vi "Live_Camram_Example_IMAQ.vi"() -> ()   [LabVIEW 2019]
doc: "A short program to demonstrate the fundamentals of control and image acquision with the pco.camera series. The program records a sequence of images, with \"live\" updating, until the \"StopRecording\" button is pressed. Use ctrl-H for more help on the individual controls and indicators.\n\nCopyright 2004, 2010 The Cooke Corporation."
uses:
  camera/Camera.lvclass
  pco.sdk/TimingControl/TimingControl.lvlib
panel:
  in  "Trigger":bool
  in  "data_format":T1(ring)=enum."Mono16"
  out "Image":T2(plugin-control)
  out "rawImage":u16[][](array[numeric])
  in  "Image Index":u32 max=9
  out "Recorded Images":u32
  in  "TriggerMode":T3(ring)
  in  "Quit":bool
  out "Error":errorcluster {"code" format="%x"}
  in  "Stop Record":bool
  out "Recording On":bool
  in  "roiY1":u64=2 min=1 max=1040 step=1
  in  "roiX1":u64=2 min=1 max=1392 step=1
  in  "roiY0":u64=1 min=1 max=1039 step=1
  in  "roiX0":u64=1 min=1 max=1391 step=1
  out "Image Height":u64
  out "Image Width":u64
  in  "segment":u16=1 caption="Segment" min=1 max=4
  in  "Exposure Time [s]":dbl=0.010000000000000002 min=1e-06 max=60.0 step=0.001
  # "This example demonstrates recording with live view for cameras with internal memory. \nDuring record, the latest transfered image is shown, after record is stopped, the images insisde the camera's ram can be addressed by index.\nNote that this example will not be fail save, i.e. doesnt react on errors, just handles them forward to the end\n\nUsage:\nSelect your required segment you want to record to, data format and the camera setup before you start the program.\nOnce started, the camera class will be initialized and images will be recorded and displayed automatically\nYou can stop the images by pressing stop record.\nAfter stopped, the image at the selected index will be read from the camera's RAM\nTo finish the program click on quit application, this will force an exit of the camera class\nYou can change your required ROI after and also during the record."
  # "pco.labview"
  # "Camera Setup"
  # "Recording Control"
  # "Parameters for image readout"
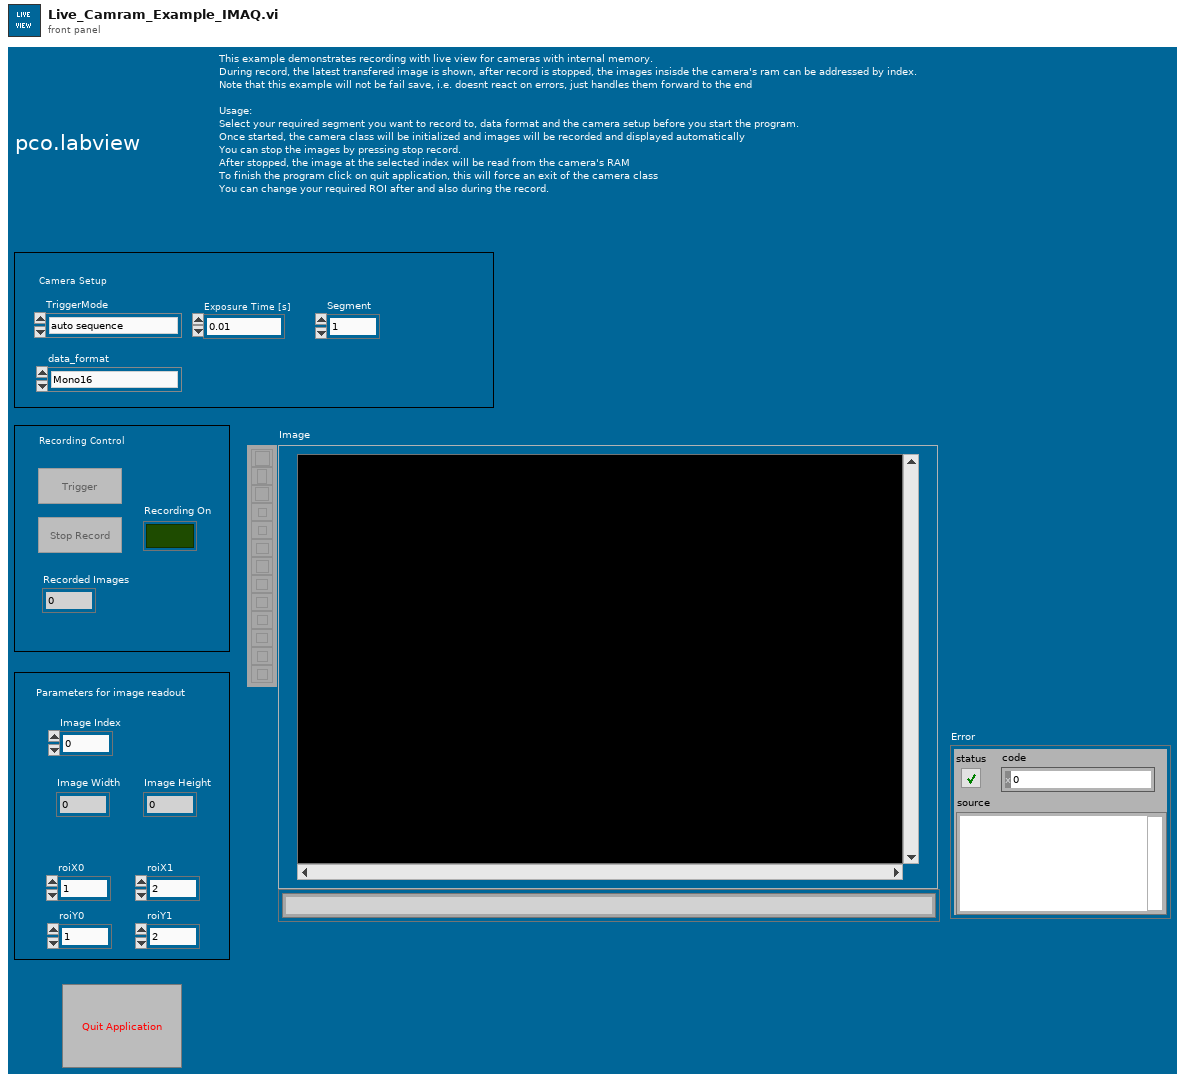
[diagram p1: front panel]
types:
  T1 = enum16{"Undefined", "Mono8", "Mono16", "BGRA8", "RGBA8", "BGRA16", "RGBA16", "CompressedMono8"}
  T2 = typedef "IMAQ Image.ctl" = refnum<image>
  T3 = enum16{"auto sequence", "software trigger", "external exposure start", "external exposure control"}
  T4 = enum16{"sequence", "sequence non blocking", "ring buffer", "fifo", "tif", "multitif", "pcoraw", "b16", "dicom", "multidicom", "camram_ring", "camram_segment"}
  T5 = enum8{"Enabled", "Disabled", "Disabled and Grayed Out"}
  T6 = cluster{"serial":u32, "type":u16, "sub_type":u16, "interface_type":u16, "bit_resolution":u16, "min_exposure_time_s":dbl, "max_exposure_time_s":dbl, "min_exposure_step_s":dbl, "min_delay_time_s":dbl, "max_delay_time_s":dbl, "min_delay_step_s":dbl, "min_width":u64, "min_height":u64, "max_width":u64, "max_height":u64, "roi_step_horz":u64, "roi_step_vert":u64, "roi_symmetric_horz":bool, "roi_symmetric_vert":bool, "has_timestamp_mode":bool, "has_timestamp_mode_ascii_only":bool, "pixelrate_vec":u32[], "conversion_factor_vec":sgl[], "has_trigger_mode_extexpctrl":bool, "has_acquire_mode":bool, "has_ext_acquire_mode":bool, "has_metadata_mode":bool, "has_ram":bool, "binning_horz_vec":u16[], "binning_vert_vec":u16[], "has_average_binning":bool, "pixel_format_vec":u32[]}
  T7 = typedef "Image Type" = u32
  T8 = cluster{"wSignalNum":u16, "wEnabled":u16, "wType":u16, "wPolarity":u16, "wFilterSetting":u16, "wSelected":u16, "dwParameter":u32[], "dwSignalFunctionality":u32[]}
  T9 = typedef "Camera.lvclass/binning.ctl" = cluster{"vert":u16, "horz":u16, "mode":u16}
  T10 = cluster{"exposure_time_s":dbl, "delay_time_s":dbl, "roi":cluster{"x0":u64, "y0":u64, "x1":u64, "y1":u64}, "timestamp_mode":u16, "pixelrate":u32, "conversion_factor":sgl, "trigger_mode":u16, "acquire_mode":u16, "acquire_sequence_number":u32, "metadata_mode":u16, "noisefilter_mode":u16, "pixel_format":u32, "binning":T9, "auto_exposure":cluster{"region":u16, "min_exposure_s":dbl, "max_exposure_s":dbl}}
  T11 = cluster{"Plane 4 (alpha)":u16, "Plane 1 (Red)":u16, "Plane 2 (Green)":u16, "Plane 3 (Blue)":u16}[][]
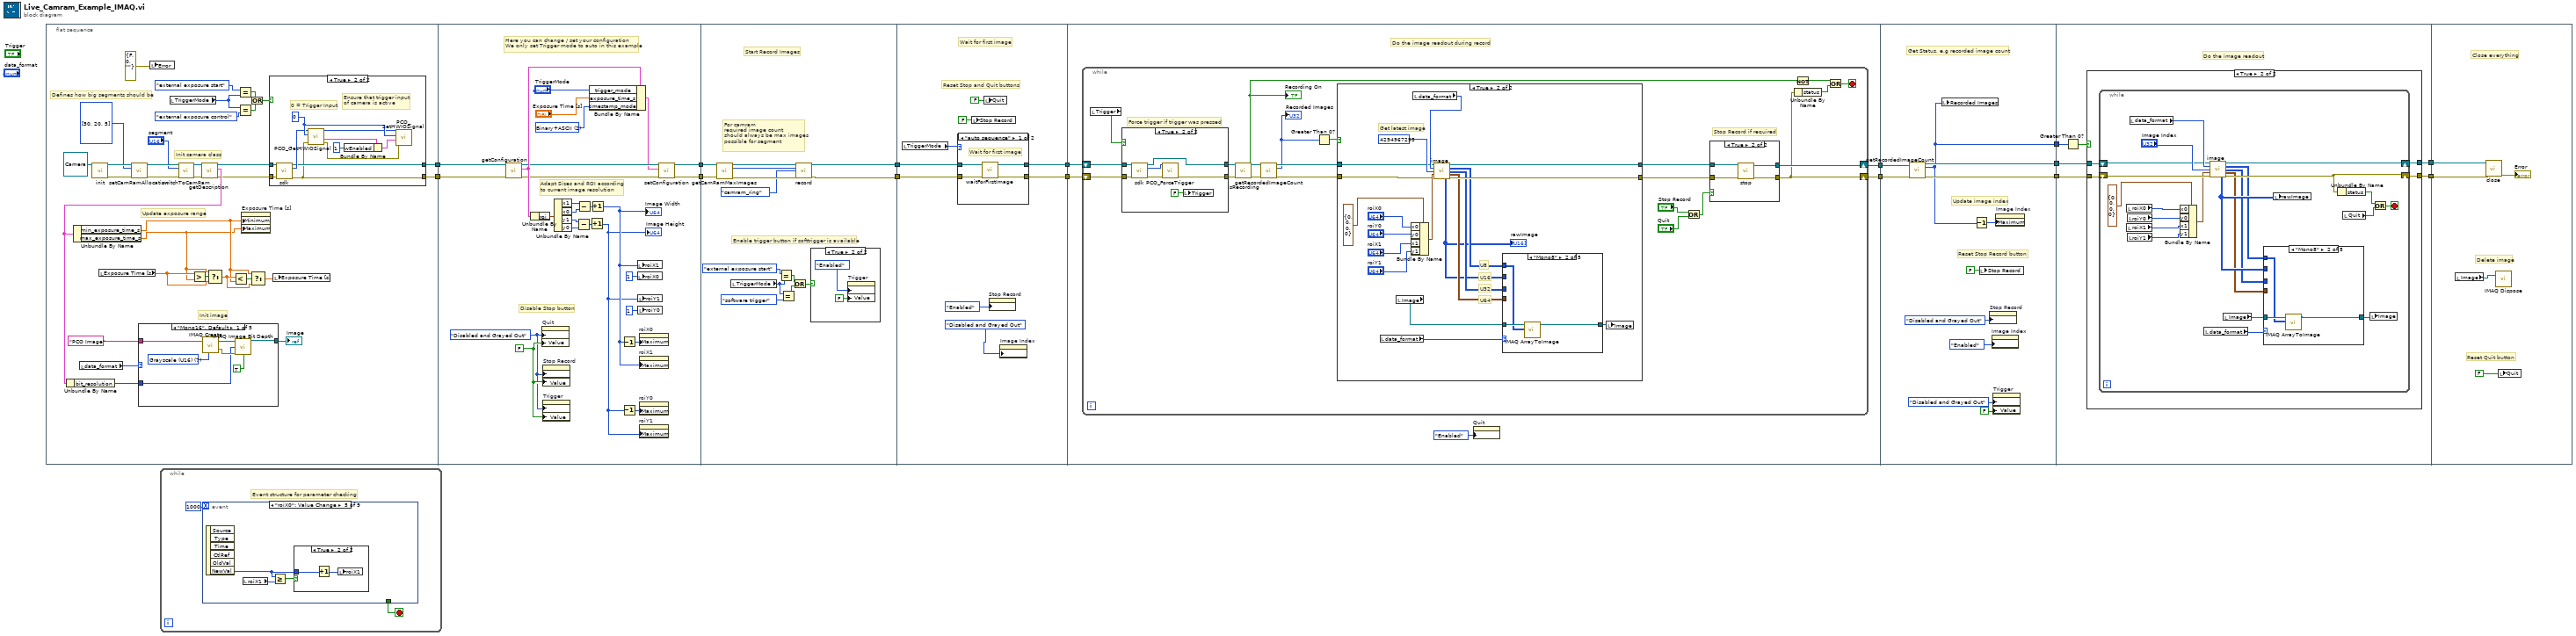
[diagram p0: block diagram]
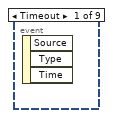
[diagram p2: hidden frame]
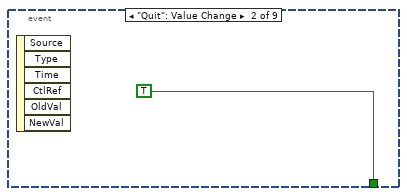
[diagram p3: hidden frame]
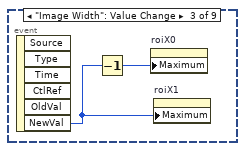
[diagram p4: hidden frame]
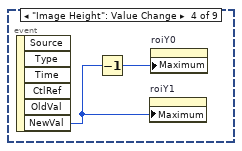
[diagram p5: hidden frame]
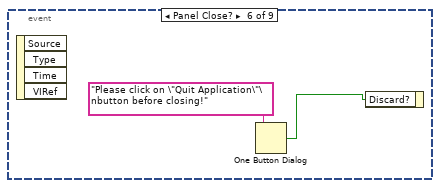
[diagram p7: hidden frame]
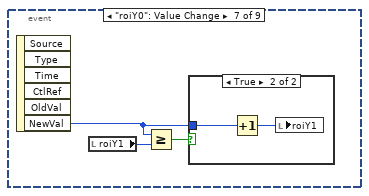
[diagram p8: hidden frame]
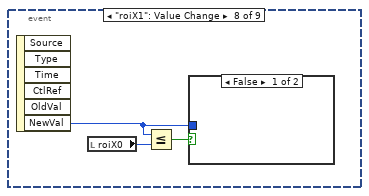
[diagram p10: hidden frame]
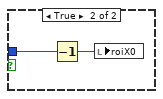
[diagram p11: hidden frame]
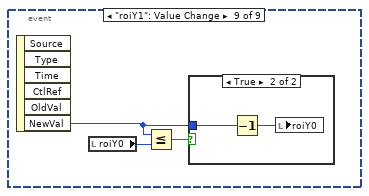
[diagram p12: hidden frame]
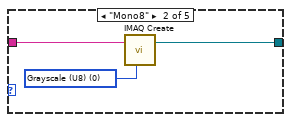
[diagram p15: hidden frame]
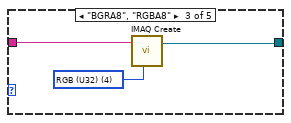
[diagram p16: hidden frame]
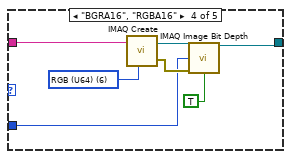
[diagram p17: hidden frame]
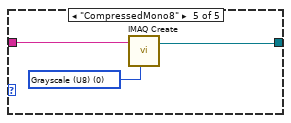
[diagram p18: hidden frame]
diagram:
  n1 = flat-sequence {
    tunnel: [w22] -> w7
    tunnel: [w23] -> w1
    tunnel: [w88] -> w15
    tunnel: [w91] -> w14
    tunnel: w7 -> [w87]
    tunnel: w1 -> [w86]
    tunnel: [w116] -> w9
    tunnel: [w117] -> w8
    tunnel: w14 -> [w114]
    tunnel: w15 -> [w115]
    tunnel: w9 -> [w130]
    tunnel: w8 -> [w131]
    tunnel: [w129] -> w13
    tunnel: [w127] -> w3
    tunnel: w13 -> [w145]
    tunnel: [w143] -> w12
    tunnel: [w142] -> w6
    tunnel: w3 -> [w141]
    tunnel: w12 -> [w227]
    tunnel: [w226] -> w11
    tunnel: w6 -> [w221]
    tunnel: [w220] -> w5
    tunnel: [w219] -> w2
    tunnel: w11 -> [w235]
    tunnel: [w234] -> w10
    tunnel: w5 -> [w233]
    tunnel: [w232] -> w4
    tunnel: w2 -> [w230]
    tunnel: w10 -> [w282]
    tunnel: w4 -> [w280]
    frame #0 {
      # "Defines how big segments should be"
      # "Init image"
      # "Init camera class"
      # "Update exposure range"
      n2 = local read "data_format"() -> (w36:T1)
      n3 = call-dynamic "init.vi"("Camera in"=refnum<class "Camera.lvclass"> refnum) -> ("Camera out"=w31:refnum<class "Camera.lvclass">, "error out"=w30:errorcluster)  [unwired: 8 in]
      n4 = local read "Exposure Time [s]"() -> (w46:dbl)
      n5 = call-dynamic "setCamRamAllocation.vi"("Camera in"=w31, "percents"=u32[] [50, 20, 5], "error in (no error)"=w30) -> ("Camera out"=w33:refnum<class "Camera.lvclass">, "error out"=w32:errorcluster)  [unwired: 11 in]
      n6 = local write "Error"(errorcluster {"status"=FALSE, "code"=0, "source"=""} ("error IO")) -> ()
      n7 = local read "TriggerMode"() -> (w16:T3)
      n8 = call-dynamic "switchToCamRam.vi"("Camera in"=w33, "segment"="segment", "error in (no error)"=w32) -> ("Camera out"=w28:refnum<class "Camera.lvclass">, "error out"=w29:errorcluster)  [unwired: 11 in]
      n9 = call-dynamic "getDescription.vi"("error in (no error)"=w29, "Camera in"=w28) -> ("error out"=w24:errorcluster, "description"=w35:T6, "Camera out"=w25:refnum<class "Camera.lvclass">)  [unwired: 7 in]
      n10 = Unbundle By Name(w35) -> ("bit_resolution"=w34:u16)
      n11 = Unbundle By Name(w35) -> ("min_exposure_time_s"=w38:dbl, "max_exposure_time_s"=w37:dbl)
      n12 = case shown="\"Mono16\", Default" w36 {
        tunnel: "PCO Image" ("Image Name") -> [w66 w70 w72 w79 w82]
        tunnel: [w62 w68 w71 w76 w81] -> w39
        tunnel: w34 -> [w61 _ _ w74 _]
        frame "Mono16", Default {
          w67 = T7 7 items=["Grayscale (U8)", "Grayscale (I16)", "Grayscale (SGL)", "Complex (CSG)", "RGB (U32)", "HSL (U32)", "RGB (U64)", "Grayscale (U16)"] ("Image Type")
          n13 = call "IMAQ Create"("Image Name"=w66, "Image Type"=w67) -> ("New Image"=w64:T2, "error out"=w63:errorcluster)  [unwired: 3 in]
          n14 = call "IMAQ Image Bit Depth"("Image"=w64, "Bit Depth (0)"=w61, "error in (no error)"=w63, "Get/Set Bit Depth? (Set)"=TRUE) -> ("Image Out"=w62:T2)  [unwired: 9 in, 2 out]
        }
        frame "Mono8" {
          w69 = T7 0 items=["Grayscale (U8)", "Grayscale (I16)", "Grayscale (SGL)", "Complex (CSG)", "RGB (U32)", "HSL (U32)", "RGB (U64)", "Grayscale (U16)"] ("Image Type")
          n15 = call "IMAQ Create"("Image Name"=w70, "Image Type"=w69) -> ("New Image"=w68:T2)  [unwired: 3 in, 1 out]
        }
        frame "BGRA8", "RGBA8" {
          w73 = T7 4 items=["Grayscale (U8)", "Grayscale (I16)", "Grayscale (SGL)", "Complex (CSG)", "RGB (U32)", "HSL (U32)", "RGB (U64)", "Grayscale (U16)"] ("Image Type")
          n16 = call "IMAQ Create"("Image Name"=w72, "Image Type"=w73) -> ("New Image"=w71:T2)  [unwired: 3 in, 1 out]
        }
        frame "BGRA16", "RGBA16" {
          w80 = T7 6 items=["Grayscale (U8)", "Grayscale (I16)", "Grayscale (SGL)", "Complex (CSG)", "RGB (U32)", "HSL (U32)", "RGB (U64)", "Grayscale (U16)"] ("Image Type")
          n17 = call "IMAQ Create"("Image Name"=w79, "Image Type"=w80) -> ("New Image"=w77:T2, "error out"=w75:errorcluster)  [unwired: 3 in]
          n18 = call "IMAQ Image Bit Depth"("Image"=w77, "Bit Depth (0)"=w74, "error in (no error)"=w75, "Get/Set Bit Depth? (Set)"=TRUE) -> ("Image Out"=w76:T2)  [unwired: 9 in, 2 out]
        }
        frame "CompressedMono8" {
          w83 = T7 0 items=["Grayscale (U8)", "Grayscale (I16)", "Grayscale (SGL)", "Complex (CSG)", "RGB (U32)", "HSL (U32)", "RGB (U64)", "Grayscale (U16)"] ("Image Type")
          n19 = call "IMAQ Create"("Image Name"=w82, "Image Type"=w83) -> ("New Image"=w81:T2)  [unwired: 3 in, 1 out]
        }
      }
      "Image" <- w39
      n20 = Greater?(x=w46, y=w37) -> (0:w47:bool)
      n21 = Select(t=w37, s=w47, f=w46) -> (s? t:f=w44:dbl)
      n22 = Less?(x=w44, y=w38) -> (x < y?=w45:bool)
      n23 = Equal?(x=T3."external exposure start" ("TriggerMode"), y=w16) -> (x = y?=w20:bool)
      n24 = Equal?(x=w16, y=T3."external exposure control" ("TriggerMode")) -> (x = y?=w19:bool)
      n25 = property on="Exposure Time [s]" class="DigNum (strict)"("Minimum"=w38, "Maximum"=w37) -> ()  [unwired: 2 in, 2 out]
      n26 = Or(x=w20, y=w19) -> (x .or. y?=w17:bool)
      n27 = Select(t=w38, s=w45, f=w44) -> (s? t:f=w43:dbl)
      n28 = case shown="True" w17 {
        tunnel: w25 -> [w49 w53]
        tunnel: w24 -> [w48 w52]
        tunnel: [w48 w50] -> w23
        tunnel: [w49 w51] -> w22
        frame False {
        }
        frame True {
          w58 = u16 0 ("wSignalNum")
          # "0 = Trigger Input"
          # "Ensure that trigger input\nof camera is active"
          n29 = call-dynamic "sdk.vi"("Camera in"=w53, "error in (no error)"=w52) -> ("Camera out"=w51:refnum<class "Camera.lvclass">, "sdk"=w54:u64, "error out"=w50:errorcluster)  [unwired: 11 in]
          n30 = call "PCO_GetHWIOSignal.vi"("error in (no error)"=w50, "wSignalNum"=w58, "ph"=w54) -> ("error out"=w56:errorcluster, "strSignal"=w60:T8, "ph out"=w55:u64)  [unwired: 5 in, 1 out]
          n31 = Bundle By Name(cluster=w60, "wEnabled"=u16 1) -> (w57:T8)
          n32 = call "PCO_SetHWIOSignal.vi"("error in (no error)"=w56, "strSignal"=w57, "wSignalNum"=w58, "ph"=w55) -> ()  [unwired: 5 in, 3 out]
        }
      }
      n33 = local write "Exposure Time [s]"(w43) -> ()
    }
    frame #1 {
      w97 = u16 2 items=["OFF", "Binary", "Binary+ASCII", "ASCII"] ("wTimeStampMode")
      w85 = FALSE ("Stop")
      w84 = T5."Disabled and Grayed Out" ("Disabled")
      # "Disable Stop button"
      # "Adapt Sizes and ROI according\nto current image resolution"
      # "Here you can change / set your configuration\nWe only set Trigger mode to auto in this example"
      n34 = call-dynamic "getConfiguration.vi"("error in (no error)"=w86, "Camera in"=w87) -> ("error out"=w92:errorcluster, "configuration"=w102:T10, "Camera out"=w94:refnum<class "Camera.lvclass">)  [unwired: 7 in]
      n35 = Unbundle By Name(w102) -> ("roi"=w103:cluster{"x0":u64, "y0":u64, "x1":u64, "y1":u64})
      n36 = property on="Quit" class="Bool (strict)"("DisabledEnum"=w84, "Value"=w85) -> ()  [unwired: 2 in, 2 out]
      n37 = property on="Stop Record" class="Bool (strict)"("DisabledEnum"=w84, "Value"=w85) -> ()  [unwired: 2 in, 2 out]
      n38 = property on="Trigger" class="Bool (strict)"("DisabledEnum"=w84, "Value"=w85) -> ()  [unwired: 2 in, 2 out]
      n39 = Unbundle By Name(w103) -> ("x1"=w105:u64, "x0"=w104:u64, "y1"=w107:u64, "y0"=w106:u64)
      n40 = Subtract(x=w107, y=w106) -> (x-y=w109:u64)
      n41 = Subtract(x=w105, y=w104) -> (x-y=w108:u64)
      n42 = Bundle By Name(cluster=w102, "trigger_mode"="TriggerMode", "exposure_time_s"="Exposure Time [s]", "timestamp_mode"=w97) -> (w93:T10)
      n43 = Increment(x=w109) -> (x+1=w89:u64)
      "Image Height" <- w89
      n44 = Increment(x=w108) -> (x+1=w90:u64)
      "Image Width" <- w90
      n45 = Decrement(x=w90) -> (x-1=w100:u64)
      n46 = Decrement(x=w89) -> (x-1=w101:u64)
      n47 = local write "roiX1"(w90) -> ()
      n48 = local write "roiX0"(u64 1 ("roiY0")) -> ()
      n49 = local write "roiY1"(w89) -> ()
      n50 = local write "roiY0"(u64 1 ("roiY0")) -> ()
      n51 = property on="roiX0" class="DigNum (strict)"("Maximum"=w100) -> ()  [unwired: 2 in, 2 out]
      n52 = property on="roiX1" class="DigNum (strict)"("Maximum"=w90) -> ()  [unwired: 2 in, 2 out]
      n53 = property on="roiY0" class="DigNum (strict)"("Maximum"=w101) -> ()  [unwired: 2 in, 2 out]
      n54 = property on="roiY1" class="DigNum (strict)"("Maximum"=w89) -> ()  [unwired: 2 in, 2 out]
      n55 = call-dynamic "setConfiguration.vi"("error in (no error)"=w92, "configuration"=w93, "Camera in"=w94) -> ("error out"=w91:errorcluster, "Camera out"=w88:refnum<class "Camera.lvclass">)  [unwired: 7 in]
    }
    frame #2 {
      # "For camram\nrequired image count \nshould always be max images\npossible for segment"
      # "Enable trigger button if softtrigger is available"
      # "Start Record Images"
      n56 = call-dynamic "getCamRamMaxImages.vi"("Camera in"=w115, "error in (no error)"=w114) -> ("Camera out"=w113:refnum<class "Camera.lvclass">, "max_images"=w111:u32, "error out"=w112:errorcluster)  [unwired: 11 in]
      n57 = local read "TriggerMode"() -> (w122:T3)
      n58 = Equal?(x=T3."external exposure start" ("TriggerMode"), y=w122) -> (x = y?=w119:bool)
      n59 = Equal?(x=w122, y=T3."software trigger" ("TriggerMode")) -> (x = y?=w118:bool)
      n60 = Or(x=w119, y=w118) -> (x .or. y?=w120:bool)
      n61 = call-dynamic "record.vi"("Camera in"=w113, "num_images"=w111, "record_mode"=T4."camram_ring", "error in (no error)"=w112) -> ("Camera out"=w117:refnum<class "Camera.lvclass">, "error out"=w116:errorcluster)  [unwired: 10 in]
      n62 = case shown="True" w120 {
        frame False {
        }
        frame True {
          n63 = property on="Trigger" class="Bool (strict)"("DisabledEnum"=T5."Enabled" ("Disabled"), "Value"=FALSE ("Trigger")) -> ()  [unwired: 2 in, 2 out]
        }
      }
    }
    frame #3 {
      # "Wait for first image"
      # "Reset Stop and Quit buttons"
      n64 = local read "TriggerMode"() -> (w126:T3)
      n65 = case shown="\"auto sequence\"" w126 {
        tunnel: w131 -> [w138 w140]
        tunnel: w130 -> [w137 w139]
        tunnel: [w136 w139] -> w129
        tunnel: [w135 w140] -> w127
        frame "auto sequence" {
          # "Wait for first image"
          n66 = call-dynamic "waitForFirstImage.vi"("error in (no error)"=w137, "Camera in"=w138) -> ("error out"=w136:errorcluster, "Camera out"=w135:refnum<class "Camera.lvclass">)  [unwired: 8 in]
        }
        frame Default {
        }
      }
      n67 = local write "Stop Record"(FALSE ("Stop Record")) -> ()
      n68 = local write "Quit"(FALSE ("Stop")) -> ()
      n69 = property on="Stop Record" class="Bool (strict)"("DisabledEnum"=T5."Enabled" ("Disabled")) -> ()  [unwired: 2 in, 2 out]
      n70 = property on="Image Index" class="DigNum (strict)"("DisabledEnum"=T5."Disabled and Grayed Out" ("Disabled")) -> ()  [unwired: 2 in, 2 out]
    }
    frame #4 {
      # "Do the image readout during record"
      n71 = while {
        shift-right: [w148] -> w143
        shift-left: w145 -> [w152]
        shift-right: [w149] -> w142
        shift-left: w141 -> [w153]
        stop <- w164 stop-if-true
        # "Force trigger if trigger was pressed"
        # "Stop Record if required"
        n72 = local read "Trigger"() -> (w154:bool)
        n73 = case shown="True" w154 {
          tunnel: w153 -> [w205 w210]
          tunnel: w152 -> [w204 w209]
          tunnel: [w205 w208] -> w151
          tunnel: [w204 w207] -> w150
          frame False {
          }
          frame True {
            n74 = call-dynamic "sdk.vi"("Camera in"=w210, "error in (no error)"=w209) -> ("Camera out"=w208:refnum<class "Camera.lvclass">, "sdk"=w211:u64, "error out"=w212:errorcluster)  [unwired: 11 in]
            n75 = call "PCO_ForceTrigger.vi"("error in (no error)"=w212, "ph"=w211) -> ("error out"=w207:errorcluster)  [unwired: 6 in, 3 out]
            n76 = local write "Trigger"(FALSE ("Trigger")) -> ()
          }
        }
        n77 = call-dynamic "isRecording.vi"("Camera in"=w151, "error in (no error)"=w150) -> ("Camera out"=w159:refnum<class "Camera.lvclass">, "recording"=w162:bool, "error out"=w158:errorcluster)  [unwired: 11 in]
        "Recording On" <- w162
        n78 = call-dynamic "getRecordedImageCount.vi"("Camera in"=w159, "error in (no error)"=w158) -> ("Camera out"=w156:refnum<class "Camera.lvclass">, "recorded_image_count"=w146:u32, "error out"=w157:errorcluster)  [unwired: 11 in]
        "Recorded Images" <- w146
        n79 = Greater Than 0?(x=w146) -> (x > 0?=w147:bool)
        n80 = case shown="True" w147 {
          tunnel: [w168 w183] -> w160
          tunnel: w157 -> [w168 w180]
          tunnel: w156 -> [w169 w171]
          tunnel: [w169 w170] -> w155
          frame False {
          }
          frame True {
            # "U64"
            # "U32"
            # "U8"
            # "U16"
            # "Get latest image"
            n81 = local read "data_format"() -> (w172:T1)
            n82 = local read "Image"() -> (w177:T2)
            n83 = Bundle By Name(cluster=cluster{"x0":u64, "y0":u64, "x1":u64, "y1":u64} {"x0"=0, "y0"=0, "x1"=0, "y1"=0} ("roi"), "x0"="roiX0", "y0"="roiY0", "x1"="roiX1", "y1"="roiY1") -> (w184:cluster{"x0":u64, "y0":u64, "x1":u64, "y1":u64})
            n84 = local read "data_format"() -> (w179:T1)
            n85 = call-dynamic "image.vi"("Camera in"=w171, "data_format"=w179, "image_index"=u32 4294967295 ("dwImgIdx"), "crop"=w184, "error in (no error)"=w180) -> ("Camera out"=w170:refnum<class "Camera.lvclass">, "image (U8)"=w174:u8[][], "image (U32)"=w175:u32[][], "image (U64)"=w176:T11, "raw_image (U16)"=w173:u16[][], "error out"=w183:errorcluster)  [unwired: 2 in, 3 out]
            "rawImage" <- w173
            n86 = case shown="\"Mono8\"" w172 {
              tunnel: w177 -> [w191 w194 w197 w200 w203]
              tunnel: [w189 w192 w196 w198 w202] -> w178
              tunnel: w176 -> [_ _ _ w199 _]
              tunnel: w175 -> [_ _ w195 _ _]
              tunnel: w174 -> [_ w193 _ _ w201]
              tunnel: w173 -> [w190 _ _ _ _]
              frame "Mono16", Default {
                n87 = call "IMAQ ArrayToImage"("Image Pixels (U16)"=w190, "Image"=w191) -> ("Image Out"=w189:T2)  [unwired: 8 in, 1 out]
              }
              frame "Mono8" {
                n88 = call "IMAQ ArrayToImage"("Image Pixels (U8)"=w193, "Image"=w194) -> ("Image Out"=w192:T2)  [unwired: 8 in, 1 out]
              }
              frame "BGRA8", "RGBA8" {
                n89 = call "IMAQ ArrayToColorImage"("Image Pixels (U32)"=w195, "Image"=w197) -> ("Image Out"=w196:T2)  [unwired: 3 in, 1 out]
              }
              frame "BGRA16", "RGBA16" {
                n90 = call "IMAQ ArrayToColorImage"("Image"=w200, "Image Pixels (U64)"=w199) -> ("Image Out"=w198:T2)  [unwired: 3 in, 1 out]
              }
              frame "CompressedMono8" {
                n91 = call "IMAQ ArrayToImage"("Image Pixels (U8)"=w201, "Image"=w203) -> ("Image Out"=w202:T2)  [unwired: 8 in, 1 out]
              }
            }
            n92 = local write "Image"(w178) -> ()
          }
        }
        n93 = Or(x="Stop Record", y="Quit") -> (x .or. y?=w165:bool)
        n94 = case shown="True" w165 {
          tunnel: w160 -> [w214 w215]
          tunnel: [w213 w217] -> w149
          tunnel: [w214 w218] -> w148
          tunnel: w155 -> [w213 w216]
          frame False {
          }
          frame True {
            n95 = call-dynamic "stop.vi"("error in (no error)"=w215, "Camera in"=w216) -> ("error out"=w218:errorcluster, "Camera out"=w217:refnum<class "Camera.lvclass">)  [unwired: 8 in]
          }
        }
        n96 = Unbundle By Name(w148) -> ("status"=w163:bool)
        n97 = Not(x=w162) -> (.not. x?=w161:bool)
        n98 = Or(x=w161, y=w163) -> (x .or. y?=w164:bool)
      }
      n99 = property on="Quit" class="Bool (strict)"("DisabledEnum"=T5."Enabled" ("Disabled")) -> ()  [unwired: 2 in, 2 out]
    }
    frame #5 {
      # "Update image index"
      # "Reset Stop Record button"
      # "Get Status, e.g recorded image count"
      n100 = call-dynamic "getRecordedImageCount.vi"("Camera in"=w221, "error in (no error)"=w227) -> ("Camera out"=w220:refnum<class "Camera.lvclass">, "recorded_image_count"=w219:u32, "error out"=w226:errorcluster)  [unwired: 11 in]
      n101 = local write "Recorded Images"(w219) -> ()
      n102 = Decrement(x=w219) -> (x-1=w224:u32)
      n103 = local write "Stop Record"(FALSE ("Stop Record")) -> ()
      n104 = property on="Stop Record" class="Bool (strict)"("DisabledEnum"=T5."Disabled and Grayed Out" ("Disabled")) -> ()  [unwired: 2 in, 2 out]
      n105 = property on="Image Index" class="DigNum (strict)"("DisabledEnum"=T5."Enabled" ("Disabled")) -> ()  [unwired: 2 in, 2 out]
      n106 = property on="Trigger" class="Bool (strict)"("DisabledEnum"=T5."Disabled and Grayed Out" ("Disabled"), "Value"=FALSE ("Trigger")) -> ()  [unwired: 2 in, 2 out]
      n107 = property on="Image Index" class="DigNum (strict)"("Maximum"=w224) -> ()  [unwired: 2 in, 2 out]
    }
    frame #6 {
      # "Do the image readout"
      n108 = Greater Than 0?(x=w230) -> (x > 0?=w231:bool)
      n109 = case shown="True" w231 {
        tunnel: w235 -> [w236 w241]
        tunnel: [w236 w240] -> w234
        tunnel: w233 -> [w237 w239]
        tunnel: [w237 w238] -> w232
        frame False {
        }
        frame True {
          n110 = while {
            shift-right: [w255] -> w240
            shift-left: w241 -> [w263]
            shift-right: [w242] -> w238
            shift-left: w239 -> [w243]
            stop <- w257 stop-if-true
            n111 = local read "roiX0"() -> (w253:u64)
            n112 = local read "roiX1"() -> (w261:u64)
            n113 = local read "roiY0"() -> (w254:u64)
            n114 = local read "roiY1"() -> (w260:u64)
            n115 = local read "data_format"() -> (w251:T1)
            n116 = Bundle By Name(cluster=cluster{"x0":u64, "y0":u64, "x1":u64, "y1":u64} {"x0"=0, "y0"=0, "x1"=0, "y1"=0} ("roi"), "x0"=w253, "y0"=w254, "x1"=w261, "y1"=w260) -> (w262:cluster{"x0":u64, "y0":u64, "x1":u64, "y1":u64})
            n117 = local read "data_format"() -> (w244:T1)
            n118 = call-dynamic "image.vi"("Camera in"=w243, "data_format"=w251, "image_index"="Image Index", "crop"=w262, "error in (no error)"=w263) -> ("Camera out"=w242:refnum<class "Camera.lvclass">, "image (U8)"=w247:u8[][], "image (U32)"=w246:u32[][], "image (U64)"=w245:T11, "raw_image (U16)"=w248:u16[][], "error out"=w255:errorcluster)  [unwired: 2 in, 3 out]
            n119 = local read "Image"() -> (w249:T2)
            n120 = case shown="\"Mono8\"" w244 {
              tunnel: w249 -> [w266 w269 w272 w275 w278]
              tunnel: [w264 w267 w271 w273 w277] -> w250
              tunnel: w245 -> [_ _ _ w274 _]
              tunnel: w246 -> [_ _ w270 _ _]
              tunnel: w247 -> [_ w268 _ _ w276]
              tunnel: w248 -> [w265 _ _ _ _]
              frame "Mono16", Default {
                n121 = call "IMAQ ArrayToImage"("Image Pixels (U16)"=w265, "Image"=w266) -> ("Image Out"=w264:T2)  [unwired: 8 in, 1 out]
              }
              frame "Mono8" {
                n122 = call "IMAQ ArrayToImage"("Image Pixels (U8)"=w268, "Image"=w269) -> ("Image Out"=w267:T2)  [unwired: 8 in, 1 out]
              }
              frame "BGRA8", "RGBA8" {
                n123 = call "IMAQ ArrayToColorImage"("Image Pixels (U32)"=w270, "Image"=w272) -> ("Image Out"=w271:T2)  [unwired: 3 in, 1 out]
              }
              frame "BGRA16", "RGBA16" {
                n124 = call "IMAQ ArrayToColorImage"("Image"=w275, "Image Pixels (U64)"=w274) -> ("Image Out"=w273:T2)  [unwired: 3 in, 1 out]
              }
              frame "CompressedMono8" {
                n125 = call "IMAQ ArrayToImage"("Image Pixels (U8)"=w276, "Image"=w278) -> ("Image Out"=w277:T2)  [unwired: 8 in, 1 out]
              }
            }
            n126 = local write "rawImage"(w248) -> ()
            n127 = Unbundle By Name(w255) -> ("status"=w258:bool)
            n128 = local read "Quit"() -> (w259:bool)
            n129 = local write "Image"(w250) -> ()
            n130 = Or(x=w258, y=w259) -> (x .or. y?=w257:bool)
          }
        }
      }
    }
    frame #7 {
      # "Delete image"
      # "Close everything"
      # "Reset Quit button"
      n131 = local read "Image"() -> (w279:T2)
      n132 = call-dynamic "close.vi"("error in (no error)"=w282, "Camera in"=w280) -> ("error out"=→"Error":errorcluster)  [unwired: 9 in]
      n133 = call "IMAQ Dispose"("Image"=w279) -> ()  [unwired: 5 in, 1 out]
      n134 = local write "Quit"(FALSE ("Stop Record")) -> ()
    }
  }
  n135 = while {
    stop <- w284 stop-if-true
    # "Event structure for parameter checking"
    n136 = event shown="[4] \"roiX0\": Value Change" {
      selector: _ -> [_ _ _ _ _ _ _ _ _]
      dyn-events: _ -> [_ _ _ _ _ _ _ _ _]
      timeout: 1000 -> [_ _ _ _ _ _ _ _ _]
      tunnel: [_ TRUE _ _ _ _ _ _ _] -> w284
      event Timeout {
        n137 = event-data() -> ()  [unwired: 1 in, 3 out]
      }
      event "Quit": Value Change {
        n138 = event-data() -> ()  [unwired: 1 in, 6 out]
      }
      event "Image Width": Value Change {
        n139 = event-data() -> ("NewVal"=w287:u64)  [unwired: 1 in, 5 out]
        n140 = Decrement(x=w287) -> (x-1=w288:u64)
        n141 = property on="roiX0" class="DigNum (strict)"("Maximum"=w288) -> ()  [unwired: 2 in, 2 out]
        n142 = property on="roiX1" class="DigNum (strict)"("Maximum"=w287) -> ()  [unwired: 2 in, 2 out]
      }
      event "Image Height": Value Change {
        n143 = event-data() -> ("NewVal"=w289:u64)  [unwired: 1 in, 5 out]
        n144 = Decrement(x=w289) -> (x-1=w290:u64)
        n145 = property on="roiY1" class="DigNum (strict)"("Maximum"=w289) -> ()  [unwired: 2 in, 2 out]
        n146 = property on="roiY0" class="DigNum (strict)"("Maximum"=w290) -> ()  [unwired: 2 in, 2 out]
      }
      event "roiX0": Value Change {
        n147 = event-data() -> ("NewVal"=w291:u64)  [unwired: 1 in, 5 out]
        n148 = local read "roiX1"() -> (w293:u64)
        n149 = Greater Or Equal?(x=w291, y=w293) -> (x >= y?=w292:bool)
        n150 = case shown="True" w292 {
          tunnel: w291 -> [_ w295]
          frame False {
          }
          frame True {
            n151 = Increment(x=w295) -> (x+1=w294:u64)
            n152 = local write "roiX1"(w294) -> ()
          }
        }
      }
      event Panel Close? {
        n153 = event-data() -> ()  [unwired: 1 in, 4 out]
        n154 = One Button Dialog(message="Please click on \"Quit Application\"\nbutton before closing!") -> (true=w296:bool)  [unwired: 1 in]
        n155 = event-data("Discard?"=w296) -> ()  [unwired: 1 in, 1 out]
      }
      event "roiY0": Value Change {
        n156 = event-data() -> ("NewVal"=w298:u64)  [unwired: 1 in, 5 out]
        n157 = local read "roiY1"() -> (w300:u64)
        n158 = Greater Or Equal?(x=w298, y=w300) -> (x >= y?=w299:bool)
        n159 = case shown="True" w299 {
          tunnel: w298 -> [_ w302]
          frame False {
          }
          frame True {
            n160 = Increment(x=w302) -> (x+1=w301:u64)
            n161 = local write "roiY1"(w301) -> ()
          }
        }
      }
      event "roiX1": Value Change {
        n162 = event-data() -> ("NewVal"=w303:u64)  [unwired: 1 in, 5 out]
        n163 = local read "roiX0"() -> (w305:u64)
        n164 = Less Or Equal?(x=w303, y=w305) -> (x <= y?=w304:bool)
        n165 = case shown="False" w304 {
          tunnel: w303 -> [_ w307]
          frame False {
          }
          frame True {
            n166 = Decrement(x=w307) -> (x-1=w306:u64)
            n167 = local write "roiX0"(w306) -> ()
          }
        }
      }
      event "roiY1": Value Change {
        n168 = event-data() -> ("NewVal"=w308:u64)  [unwired: 1 in, 5 out]
        n169 = local read "roiY0"() -> (w310:u64)
        n170 = Less Or Equal?(x=w308, y=w310) -> (x <= y?=w309:bool)
        n171 = case shown="True" w309 {
          tunnel: w308 -> [_ w312]
          frame False {
          }
          frame True {
            n172 = Decrement(x=w312) -> (x-1=w311:u64)
            n173 = local write "roiY0"(w311) -> ()
          }
        }
      }
    }
  }
